vi "test - clear JKI String Queue Error.vi"(8 "error in (no error)":errorcluster, 11 "TestCase in":refnum<class "testcase-Basic-Function.lvclass">) -> (0 "error out":errorcluster, 3 "TestCase out":refnum<class "testcase-Basic-Function.lvclass">)   [LabVIEW 2017, in "testcase-Basic-Function.lvclass"]
uses:
  testcase-Basic-Function.lvclass
  161a5074-68cb-42ac-bbbd-290e101bf616.vi
  src/user.lib/_NEVSTOP/Communicable State Machine(CSM)/AdvanceAPI/CSM - Revert Arguments-Safe String.vi
  src/user.lib/_NEVSTOP/Communicable State Machine(CSM)/_Shared/Trim Single-line Text.vi
  src/user.lib/_NEVSTOP/Communicable State Machine(CSM)/AdvanceAPI/CSM - Make String Arguments Safe.vi
  src/user.lib/_NEVSTOP/Communicable State Machine(CSM)/AdvanceAPI/CSM - Break Down Multiple States String.vi
  src/user.lib/_NEVSTOP/Communicable State Machine(CSM)/AdvanceAPI/CSM - Compact Multiple States.vi
  src/user.lib/_NEVSTOP/Communicable State Machine(CSM)/AdvanceAPI/CSM - Keywords.vi
  <vilib>/addons/_JKI Toolkits/VI Tester/TestCase.llb/TestCase.lvclass
  src/user.lib/_NEVSTOP/Communicable State Machine(CSM)/Communicable State Machine.lvlib
  C:/Program Files (x86)/National Instruments/LabVIEW 2017/vi.lib/addons/_JKI Toolkits/VI Tester/TestCase.llb/TestCase.lvclass
panel:
  out "error in CSM":errorcluster
  in  "x":bool
  out "error for return":errorcluster
  out "State History":string
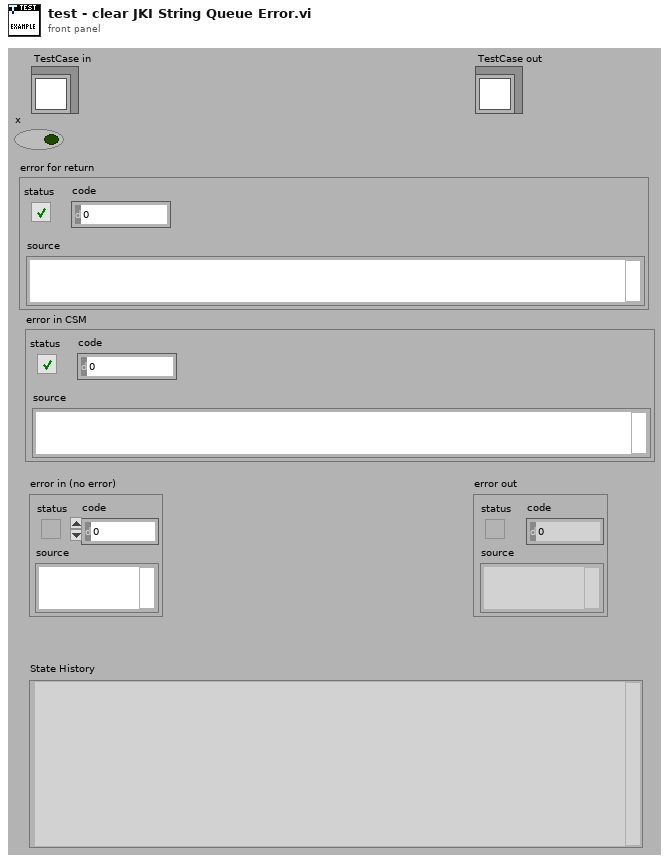
[diagram p1: front panel]
types:
  T1 = enum32{"Invalid", "Standard", "Closed", "Hidden", "Minimized", "Maximized"}
  T2 = enum32{"invalid app kind", "Development System", "Run Time System", "Student Edition", "Embedded LabVIEW", "Evaluation", "Custom"}
  T3 = typedef "Communicable State Machine.lvlib/_CSM_Response Source Message.ctl" = cluster{"‘State":string, "’Arguments":string, "’Error":errorcluster}
  T4 = cluster{"Current VI Reference":refnum<vi>, "Close Panel on Exit?":bool}
  T5 = cluster{"Core":cluster{"Current VI Reference":refnum<vi>, "Close Panel on Exit?":bool}, "Your Boolean data":bool, "Your string data":string}
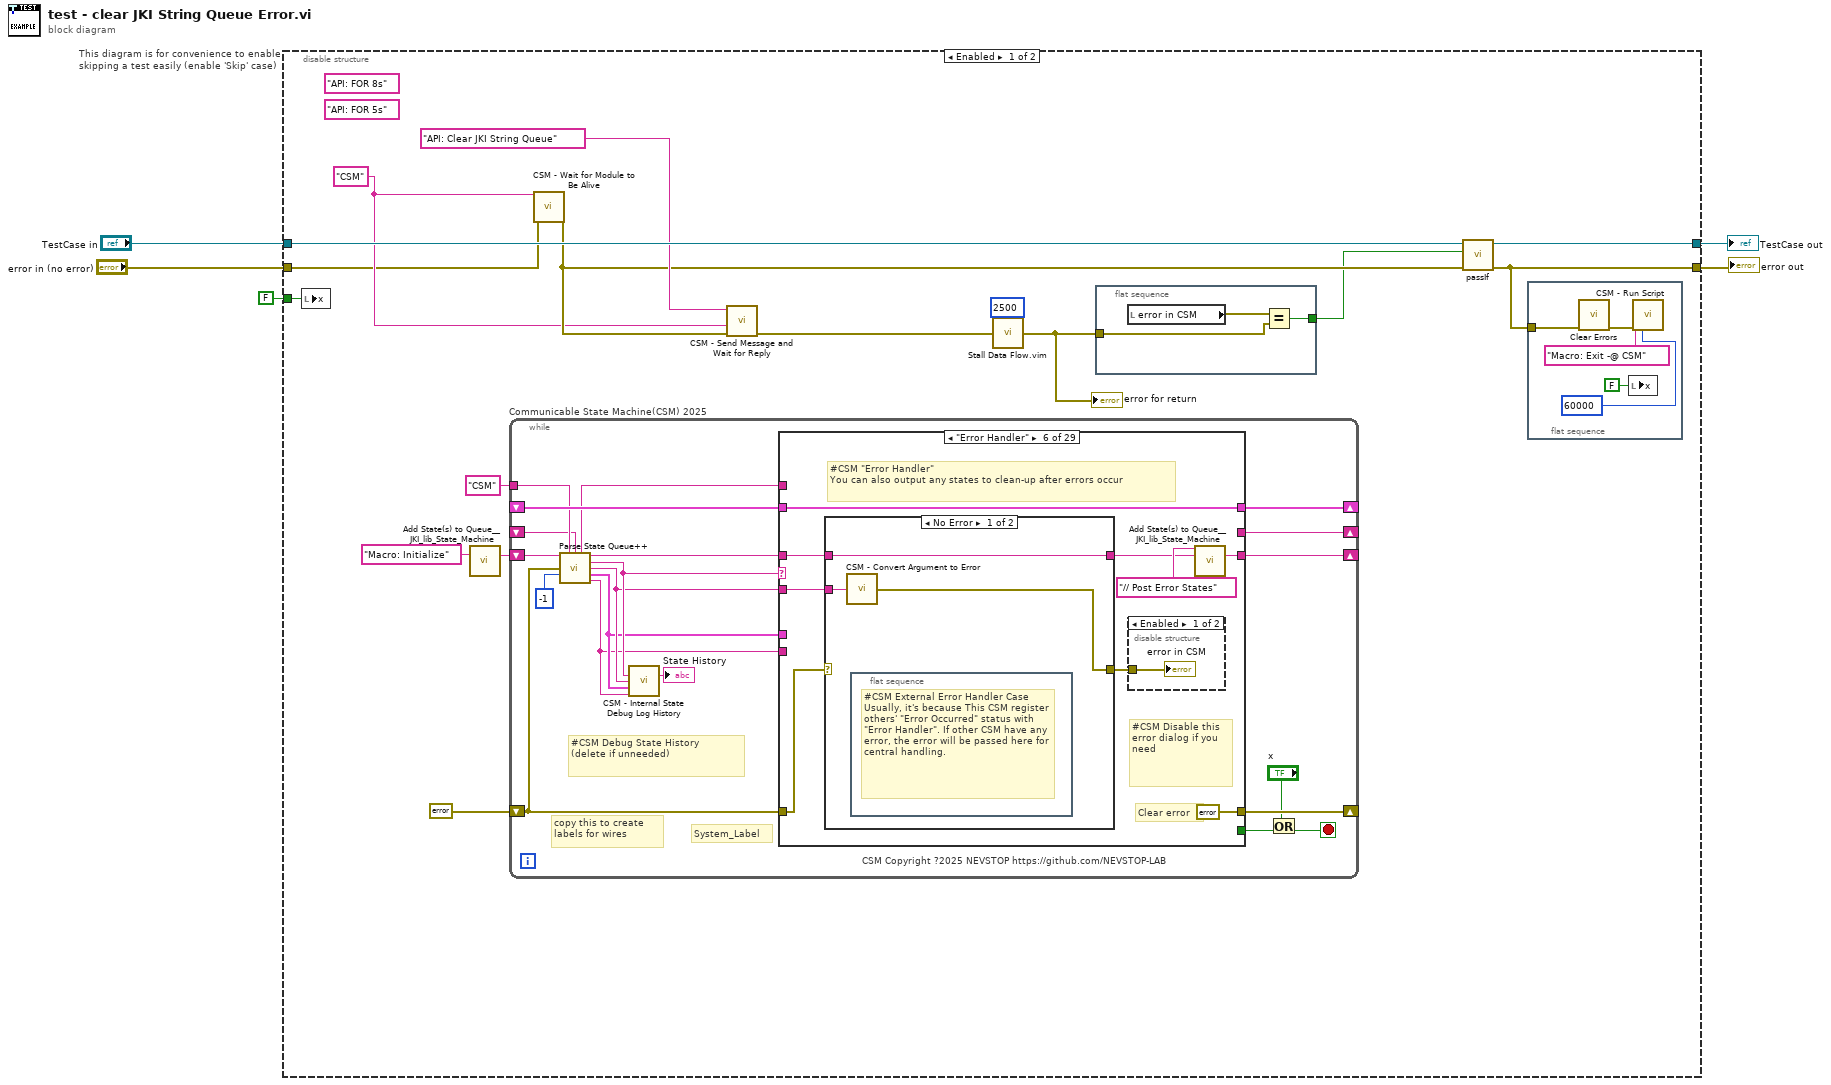
[diagram p0: block diagram]
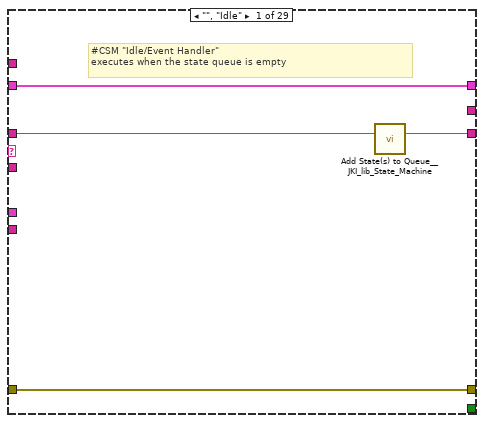
[diagram p2: hidden frame]
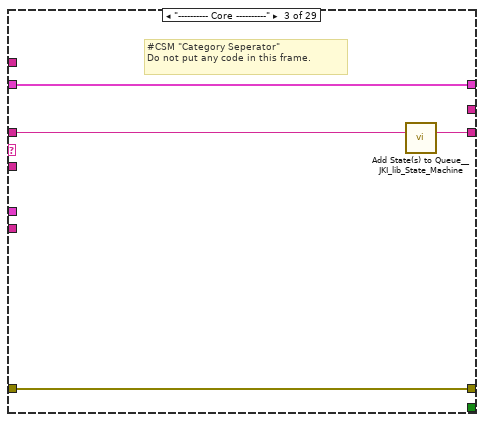
[diagram p4: hidden frame]
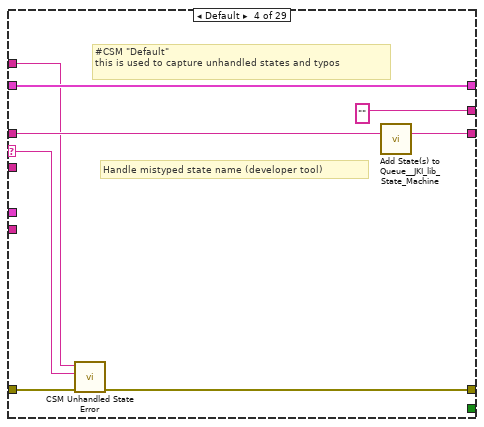
[diagram p5: hidden frame]
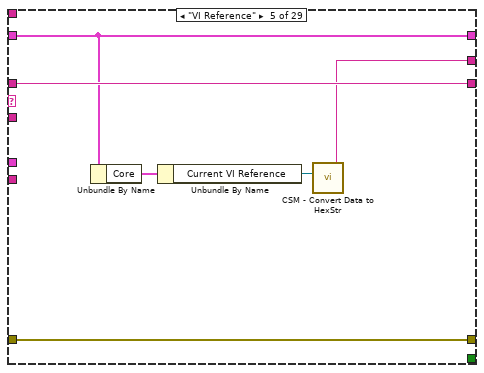
[diagram p6: hidden frame]
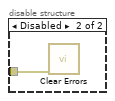
[diagram p7: hidden frame]
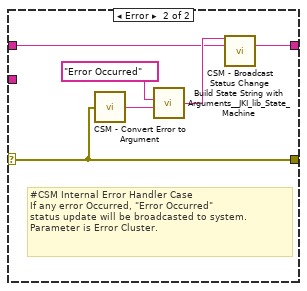
[diagram p8: hidden frame]
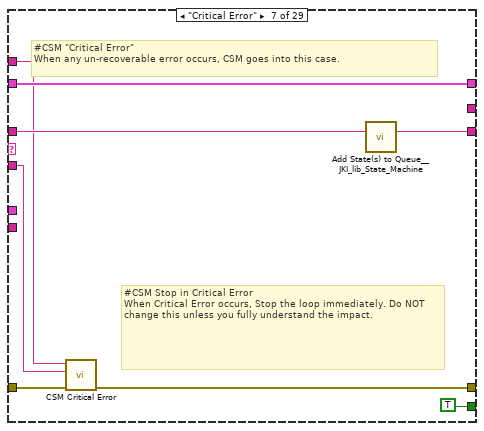
[diagram p9: hidden frame]
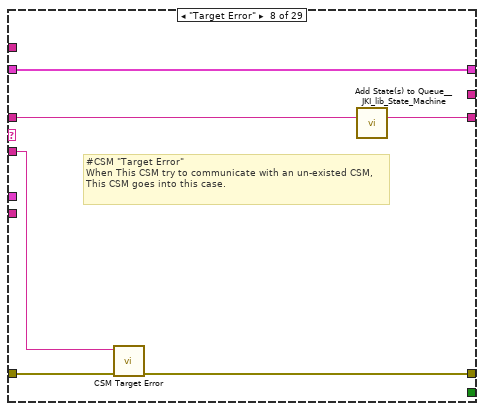
[diagram p10: hidden frame]
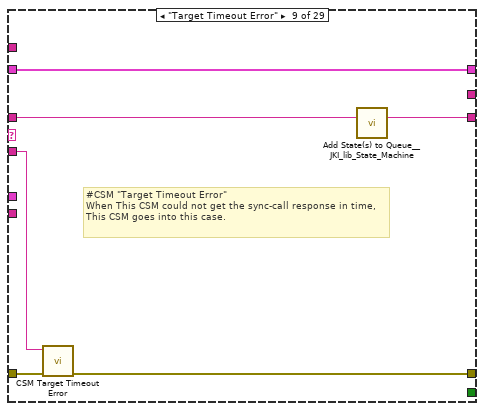
[diagram p11: hidden frame]
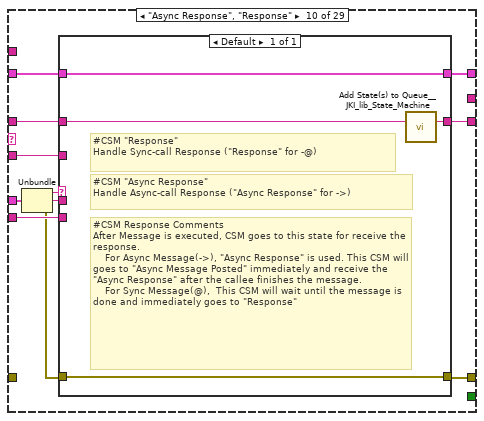
[diagram p12: hidden frame]
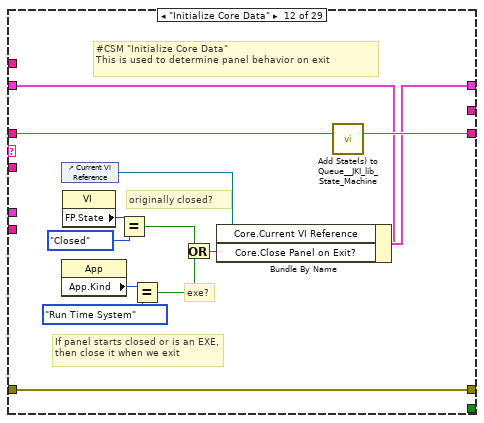
[diagram p14: hidden frame]
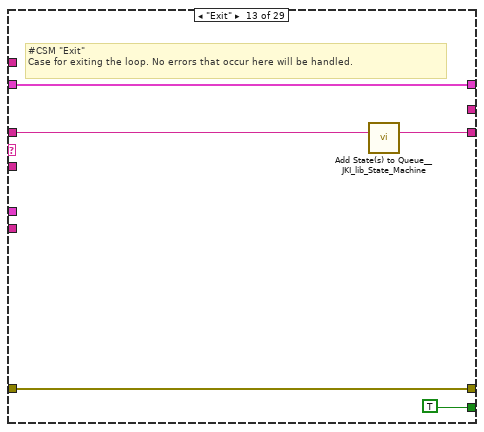
[diagram p15: hidden frame]
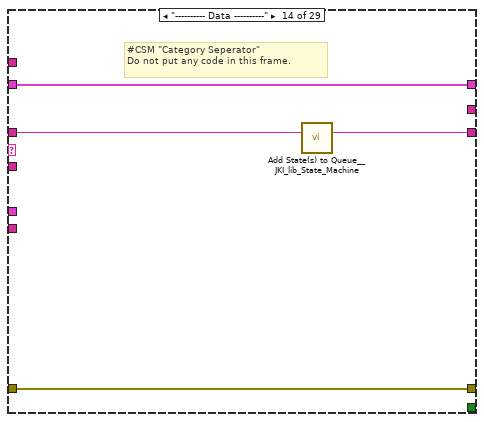
[diagram p16: hidden frame]
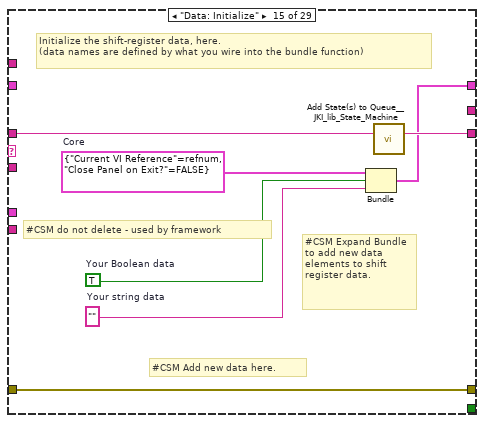
[diagram p17: hidden frame]
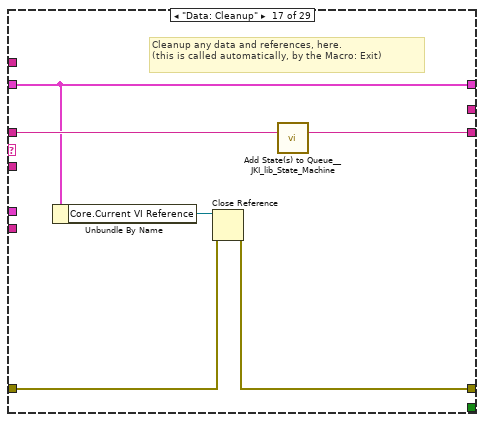
[diagram p19: hidden frame]
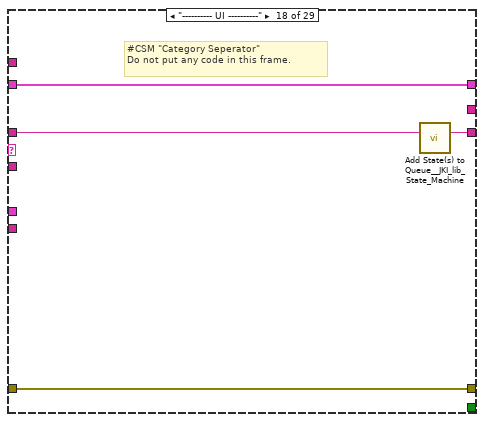
[diagram p20: hidden frame]
diagram:
  n1 = disable-structure "This diagram is for convenience to enable skipping a test easily (enable 'Skip' case)" shown="Enabled" {
    disable-tunnel: "TestCase in" -> [w15 w301]
    disable-tunnel: [w17 w299] -> w2
    disable-tunnel: [w16 w300] -> w4
    disable-tunnel: "error in (no error)" -> [w11 w298]
    disable-tunnel: FALSE ("x") -> [w8 _]
    frame Enabled {
      (unwired) "API: FOR 8s" ("State")
      (unwired) "API: FOR 5s" ("State")
      w12 = "CSM" ("Name (\"\" to Use UUID)")
      n2 = local write "x"(w8) -> ()
      n3 = call <vilib>:"Add State(s) to Queue__JKI_lib_State_Machine.vi"("State(s) in (\"\")"="Macro: Initialize" ("Init State(\"Macro: Initialize\")")) -> ("States Out"=w21:string)  [unwired: 14 in]
      n4 = while "Communicable State Machine(CSM) 2025" {
        shift-right: [w44] -> _
        shift-left: _ -> [w43]
        shift-right: [w47] -> _
        shift-left: errorcluster {"status"=FALSE, "code"=0, "source"=""} ("error out") -> [w42]
        shift-right: [w46] -> _
        shift-left: w21 -> [w48]
        tunnel: "CSM" ("Name (\"\" to Use UUID)") -> [w40]
        shift-right: [w41] -> _
        shift-left: _ -> [w34]
        stop <- w31 stop-if-true
        # "#CSM Debug State History\n(delete if unneeded)"
        # "copy this to create labels for wires"
        # "System_Label"
        # "CSM Copyright ?2025 NEVSTOP https://github.com/NEVSTOP-LAB"
        n5 = call "Parse State Queue++.vi"("State Queue"=w48, "Name (\"\" to Use UUID)"=w40, "Response Arguments"=w34, "Previous Error"=w42, "Dequeue (1 ms)"=-1 ("Timeout")) -> ("Name Used"=w35:string, "Remaining States"=w49:string, "Current State"=w39:string, "Arguments"=w38:string, "Additional Information"=w37:T3, "Source CSM"=w36:string)  [unwired: 5 in]
        n6 = call "CSM - Internal State Debug Log History.vi"("State"=w39, "Arguments (\"\")"=w38, ">> Response Source Message >>"=w37, "Source (\"\")"=w36) -> ("Debug Log"=→"State History":string)  [unwired: 11 in]
        n7 = case shown="\"Error Handler\"" w39 {
          selector: w39 -> [_ _ _ w63 _ _ _ _ _ _ _ _ _ _ _ _ _ _ _ _ _ _ _ _ _ _ _ _ _]
          tunnel: w49 -> [w50 w55 w60 w67 w73 w79 w100 w106 w112 w120 w131 w145 w150 w154 w161 w163 w170 w174 w178 w184 w199 w268 w273 w280 w282 _ w289 w293 w297]
          tunnel: w38 -> [_ _ _ _ _ w78 w96 w105 w110 w119 _ _ _ _ _ _ _ _ _ w179 w193 _ _ _ _ _ _ _ _]
          tunnel: w43 -> [w51 w54 w57 w65 w72 w82 w101 w107 w113 w122 w130 w138 w148 w151 _ w162 w165 w171 w176 w182 w195 w265 w270 w277 w281 w284 w286 w290 w294]
          tunnel: [w52 w56 w58 w61 w74 errorcluster {"status"=FALSE, "code"=0, "source"=""} ("error out") w97 w103 w109 w125 w132 w142 w147 w152 w158 w164 w166 w172 w175 w180 w196 w266 w271 w278 w283 w285 w287 w291 w295] -> w47
          tunnel: w42 -> [w52 w56 w58 w68 w74 w80 w102 w104 w111 _ w132 w142 w147 w152 w158 w164 w167 w172 w175 w181 w197 w266 w271 w278 w283 w285 w287 w291 w295]
          tunnel: [w53 w55 w59 w66 w73 w75 w99 w108 w114 w121 w131 w144 w149 w153 w160 w163 w169 w173 w177 w183 w198 w267 w272 w279 w282 _ w288 w292 w296] -> w46
          tunnel: [_ _ _ _ _ _ TRUE _ _ _ _ _ TRUE _ _ _ _ _ _ _ _ _ _ _ _ _ _ _ _] -> w45
          tunnel: [w51 w54 w57 w65 w72 w82 w101 w107 w113 w123 w130 w143 w148 w151 w159 w162 w165 w171 w176 w182 w195 w265 w270 w277 w281 w284 w286 w290 w294] -> w44
          tunnel: w36 -> [_ _ _ _ _ _ _ _ _ w117 _ _ _ _ _ _ _ _ _ _ _ _ _ _ _ _ _ _ _]
          tunnel: w37 -> [_ _ _ _ _ _ _ _ _ w124 _ _ _ _ _ _ _ _ _ _ _ _ _ _ _ _ _ _ _]
          tunnel: [_ _ _ "" w69 _ _ _ _ _ _ _ _ _ _ _ _ _ _ _ _ _ _ _ _ _ _ _ _] -> w41
          tunnel: w35 -> [_ _ _ w62 _ _ w95 _ _ _ _ _ _ _ _ _ _ _ _ _ _ _ _ _ _ _ _ _ _]
          frame "", "Idle" {
            # "#CSM \"Idle/Event Handler\"\nexecutes when the state queue is empty"
            n8 = call <vilib>:"Add State(s) to Queue__JKI_lib_State_Machine.vi"("State(s) in (\"\")"=w50) -> ("States Out"=w53:string)  [unwired: 14 in]
          }
          frame "CSM Documentation" {
            # "#CSM README FIRST\n\nCommunicable State Machine(CSM) is a LabVIEW application framework that builds upon JKI State Machine(JKISM). It follows the pattern of JKISM and extends the keywords to describe message communication between modules, including concepts such as Sync-Message, Async-Message, Subscription/Unsubscription of status - essential elements for creating reusable code modules. For more information, please visit the CSM wiki: https://nevstop-lab.github.io/CSM-Wiki/\n\nFor instructions on JKI State Machine, visit: http://jki.net/state-machine/\nFor information about CSM, visit: https://github.com/NEVSTOP-LAB"
            # "#CSM \"Documentation\"\nCase for holding CSM Documenation"
          }
          frame "---------- Core ----------" {
            # "#CSM \"Category Seperator\"\nDo not put any code in this frame."
            n9 = call <vilib>:"Add State(s) to Queue__JKI_lib_State_Machine.vi"("State(s) in (\"\")"=w60) -> ("States Out"=w59:string)  [unwired: 14 in]
          }
          frame Default {
            # "#CSM \"Default\"\nthis is used to capture unhandled states and typos"
            # "Handle mistyped state name (developer tool)"
            n10 = call "CSM Unhandled State Error.vi"("error in (no error)"=w68, "Undefined State"=w63, "CSM Name"=w62) -> ("error out"=w61:errorcluster)  [unwired: 8 in]
            n11 = call <vilib>:"Add State(s) to Queue__JKI_lib_State_Machine.vi"("State(s) in (\"\")"=w67) -> ("States Out"=w66:string)  [unwired: 14 in]
          }
          frame "VI Reference" {
            n12 = Unbundle By Name(w72) -> ("Core"=w71:T4)
            n13 = Unbundle By Name(w71) -> ("Current VI Reference"=w70:refnum<vi>)
            n14 = call "CSM - Convert Data to HexStr.vi"("Variant"=w70) -> ("HEX String (0-9,A-F)"=w69:string)  [unwired: 8 in]
          }
          frame "Error Handler" {
            # "#CSM Disable this error dialog if you need"
            # "#CSM \"Error Handler\"\nYou can also output any states to clean-up after errors occur"
            # "Clear error"
            n15 = case shown="No Error" w80 {
              selector: w80 -> [_ w89]
              tunnel: [w88 w91] -> w76
              tunnel: w79 -> [w88 w90]
              tunnel: w78 -> [w87 _]
              tunnel: [w86 w89] -> w81
              frame No Error {
                n16 = call "CSM - Convert Argument to Error.vi"("Argument"=w87) -> ("Error"=w86:errorcluster)  [unwired: 4 in]
                n17 = flat-sequence {
                  frame #0 {
                    # "#CSM External Error Handler Case\nUsually, it's because This CSM register others' \"Error Occurred\" status with \"Error Handler\". If other CSM have any error, the error will be passed here for central handling."
                  }
                }
              }
              frame Error {
                # "#CSM Internal Error Handler Case \nIf any error Occurred, \"Error Occurred\" \nstatus update will be broadcasted to system.\nParameter is Error Cluster."
                n18 = call "CSM - Convert Error to Argument.vi"("Error"=w89) -> ("Argument"=w93:string)  [unwired: 4 in]
                n19 = call <vilib>:"Build State String with Arguments__JKI_lib_State_Machine.vi"("Arguments (\"\")"=w93, "State"="Error Occurred" ("Status with Arguments")) -> ("State with Arguments"=w92:string)  [unwired: 4 in]
                n20 = call "CSM - Broadcast Status Change.vi"("Status With Arguments"=w92, "State Queue"=w90) -> ("Remaining States"=w91:string)  [unwired: 13 in]
              }
            }
            n21 = disable-structure shown="Enabled" {
              disable-tunnel: w81 -> [w84 w85]
              frame Enabled {
                "error in CSM" <- w84
              }
              frame Disabled {
                n22 = call <vilib>:"Clear Errors.vi"("error in (no error)"=w85) -> ()  [unwired: 5 in, 2 out]
              }
            }
            n23 = call <vilib>:"Add State(s) to Queue__JKI_lib_State_Machine.vi"("State(s) in Front (\"\")"="// Post Error States", "State(s) in (\"\")"=w76) -> ("States Out"=w75:string)  [unwired: 13 in]
          }
          frame "Critical Error" {
            # "#CSM Stop in Critical Error\nWhen Critical Error occurs, Stop the loop immediately. Do NOT change this unless you fully understand the impact."
            # "#CSM \"Critical Error\"\nWhen any un-recoverable error occurs, CSM goes into this case."
            n24 = call "CSM Critical Error.vi"("error in (no error)"=w102, "Arugments (As Reason)"=w96, "CSM Name"=w95) -> ("error out"=w97:errorcluster)  [unwired: 8 in]
            n25 = call <vilib>:"Add State(s) to Queue__JKI_lib_State_Machine.vi"("State(s) in (\"\")"=w100) -> ("States Out"=w99:string)  [unwired: 14 in]
          }
          frame "Target Error" {
            # "#CSM \"Target Error\"\nWhen This CSM try to communicate with an un-existed CSM, This CSM goes into this case."
            n26 = call "CSM Target Error.vi"("error in (no error)"=w104, "Arguments (As CSM Name)"=w105) -> ("error out"=w103:errorcluster)  [unwired: 9 in]
            n27 = call <vilib>:"Add State(s) to Queue__JKI_lib_State_Machine.vi"("State(s) in (\"\")"=w106) -> ("States Out"=w108:string)  [unwired: 14 in]
          }
          frame "Target Timeout Error" {
            # "#CSM \"Target Timeout Error\"\nWhen This CSM could not get the sync-call response in time, This CSM goes into this case."
            n28 = call "CSM Target Timeout Error.vi"("error in (no error)"=w111, "Arguments (As CSM Name)"=w110) -> ("error out"=w109:errorcluster)  [unwired: 9 in]
            n29 = call <vilib>:"Add State(s) to Queue__JKI_lib_State_Machine.vi"("State(s) in (\"\")"=w112) -> ("States Out"=w114:string)  [unwired: 14 in]
          }
          frame "Async Response", "Response" {
            n30 = Unbundle(w124) -> ("‘State"=w118:string, "’Arguments"=w116:string, "’Error"=w115:errorcluster)
            n31 = case shown="Default" w118 {
              tunnel: [w129] -> w125
              tunnel: w115 -> [w129]
              tunnel: [w128] -> w123
              tunnel: w122 -> [w128]
              tunnel: [w126] -> w121
              tunnel: w120 -> [w127]
              tunnel: w119 -> [_]
              tunnel: w117 -> [_]
              tunnel: w116 -> [_]
              frame Default {
                # "#CSM Response Comments\nAfter Message is executed, CSM goes to this state for receive the response.\n    For Async Message(->), \"Async Response\" is used. This CSM will goes to \"Async Message Posted\" immediately and receive the \"Async Response\" after the callee finishes the message.\n    For Sync Message(@),  This CSM will wait until the message is done and immediately goes to \"Response\""
                # "#CSM \"Async Response\"\nHandle Async-call Response (\"Async Response\" for ->)"
                # "#CSM \"Response\"\nHandle Sync-call Response (\"Response\" for -@)"
                n32 = call <vilib>:"Add State(s) to Queue__JKI_lib_State_Machine.vi"("State(s) in (\"\")"=w127) -> ("States Out"=w126:string)  [unwired: 14 in]
              }
            }
          }
          frame "Async Message Posted" {
            # "#CSM \"Async Message Posted\"\nAfter Async Message is posted (-> or ->| ), CSM goes to this state for post-action.\nYou can use Argument - State to tell which Async Message is called."
          }
          frame "Initialize Core Data" {
            # "#CSM \"Initialize Core Data\"\nThis is used to determine panel behavior on exit"
            # "originally closed?"
            # "exe?"
            # "If panel starts closed or is an EXE, then close it when we exit"
            n33 = control-ref of="Current VI Reference"() -> (w136:refnum<vi>)
            n34 = property class="App"() -> ("App.Kind"=w141:T2)  [unwired: 2 in, 2 out]
            n35 = property class="VI"() -> ("FP.State"=w135:T1)  [unwired: 2 in, 2 out]
            n36 = Equal?(x=w135, y=T1."Closed" ("Front Panel Window:State")) -> (x = y?=w133:bool)
            n37 = Equal?(x=w141, y=T2."Run Time System" ("Application:Kind")) -> (x = y?=w139:bool)
            n38 = Or(x=w133, y=w139) -> (x .or. y?=w137:bool)
            n39 = Bundle By Name(cluster=w138, "Core.Current VI Reference"=w136, "Core.Close Panel on Exit?"=w137) -> (w143:T5)
            n40 = call <vilib>:"Add State(s) to Queue__JKI_lib_State_Machine.vi"("State(s) in (\"\")"=w145) -> ("States Out"=w144:string)  [unwired: 14 in]
          }
          frame "Exit" {
            # "#CSM \"Exit\"\nCase for exiting the loop. No errors that occur here will be handled."
            n41 = call <vilib>:"Add State(s) to Queue__JKI_lib_State_Machine.vi"("State(s) in (\"\")"=w150) -> ("States Out"=w149:string)  [unwired: 14 in]
          }
          frame "---------- Data ----------" {
            # "#CSM \"Category Seperator\"\nDo not put any code in this frame."
            n42 = call <vilib>:"Add State(s) to Queue__JKI_lib_State_Machine.vi"("State(s) in (\"\")"=w154) -> ("States Out"=w153:string)  [unwired: 14 in]
          }
          frame "Data: Initialize" {
            w155 = T4 {"Current VI Reference"=refnum, "Close Panel on Exit?"=FALSE}  # Core
            w157 = TRUE  # Your Boolean data
            w156 = ""  # Your string data
            # "#CSM do not delete - used by framework"
            # "#CSM Expand Bundle to add new data elements to shift register data."
            # "#CSM Add new data here."
            # "Initialize the shift-register data, here.\n(data names are defined by what you wire into the bundle function)"
            n43 = Bundle("Core"=w155, "Your Boolean data"=w157, "Your string data"=w156) -> (w159:T5)  [unwired: 1 in]
            n44 = call <vilib>:"Add State(s) to Queue__JKI_lib_State_Machine.vi"("State(s) in (\"\")"=w161) -> ("States Out"=w160:string)  [unwired: 14 in]
          }
          frame "Data: Update Indicators" {
          }
          frame "Data: Cleanup" {
            # "Cleanup any data and references, here.\n(this is called automatically, by the Macro: Exit)"
            n45 = Unbundle By Name(w165) -> ("Core.Current VI Reference"=w168:refnum<vi>)
            n46 = Close Reference(reference=w168, error in (no error)=w167) -> (error out=w166:errorcluster)
            n47 = call <vilib>:"Add State(s) to Queue__JKI_lib_State_Machine.vi"("State(s) in (\"\")"=w170) -> ("States Out"=w169:string)  [unwired: 14 in]
          }
          frame "---------- UI ----------" {
            # "#CSM \"Category Seperator\"\nDo not put any code in this frame."
            n48 = call <vilib>:"Add State(s) to Queue__JKI_lib_State_Machine.vi"("State(s) in (\"\")"=w174) -> ("States Out"=w173:string)  [unwired: 14 in]
          }
          frame "UI: Initialize" {
            # "#CSM \"UI: Initialize\"\nInitialize the User Interface, here.\n(this is called automatically, by the Macro: Init)"
            n49 = call <vilib>:"Add State(s) to Queue__JKI_lib_State_Machine.vi"("State(s) in (\"\")"=w178) -> ("States Out"=w177:string)  [unwired: 14 in]
          }
          frame "UI: Cursor Set" {
            # "#CSM \"UI: Cursor Set\"\nSet and Unset Cursor Busy.\n(Usage: \"UI: Cursor Set >> Busy|Idle\")"
            # "Argument"
            n50 = disable-structure shown="TARGET_TYPE!=Windows" {
              disable-tunnel: w181 -> [w187 w192]
              disable-tunnel: [w186 w192] -> w180
              disable-tunnel: w179 -> [w185 _]
              frame condition #0 (active) {
                n51 = case shown="\"Idle\", Default" w185 {
                  tunnel: w187 -> [w189 w191]
                  tunnel: [w188 w190] -> w186
                  frame "Idle", Default {
                    n52 = call <vilib>:"Unset Busy.vi"("error in (no error)"=w189) -> ("error out"=w188:errorcluster)  [unwired: 10 in]
                  }
                  frame "Busy" {
                    n53 = call <vilib>:"Set Busy.vi"("error in (no error)"=w191) -> ("error out"=w190:errorcluster)  [unwired: 9 in, 1 out]
                  }
                }
              }
              frame condition #1 {
              }
            }
            n54 = call <vilib>:"Add State(s) to Queue__JKI_lib_State_Machine.vi"("State(s) in (\"\")"=w184) -> ("States Out"=w183:string)  [unwired: 14 in]
          }
          frame "UI: Front Panel State" {
            # "#CSM \"UI: Front Panel State\"\nSet Front Panel Open or Closed\n(Usage: \"UI: Front Panel State >> Open|Close\")"
            # "Argument"
            n55 = Unbundle By Name(w195) -> ("Core.Current VI Reference"=w194:refnum<vi>)
            n56 = call <vilib>:"Add State(s) to Queue__JKI_lib_State_Machine.vi"("State(s) in (\"\")"=w199) -> ("States Out"=w198:string)  [unwired: 14 in]
            n57 = case shown="\"Close\", \"Closed\"" w193 {
              tunnel: w197 -> [w205 w220 w231 w244 w257]
              tunnel: [w207 w221 w233 w246 w259] -> w196
              tunnel: w194 -> [w206 w218 w232 w245 w258]
              frame "Open", "Standard", Default {
                w200 = T1."Standard" ("State")
                n58 = property class="VI"(reference=w206, error in=w205) -> (reference out=w203:refnum<vi>, error out=w204:errorcluster, "FP.State"=w202:T1)
                n59 = Not Equal?(x=w202, y=w200) -> (x != y?=w201:bool)
                n60 = case shown="True" w201 {
                  tunnel: [w211 w213] -> w207
                  tunnel: w204 -> [w210 w213]
                  tunnel: w203 -> [w209 _]
                  tunnel: w200 -> [w208 _]
                  frame True {
                    n61 = invoke class="VI" method="FP.Open"(reference=w209, error in=w210, "Activate"=TRUE, "State"=w208) -> (error out=w211:errorcluster)  [unwired: 1 in, 4 out]
                  }
                  frame False {
                  }
                }
              }
              frame "Close", "Closed" {
                n62 = property class="VI"(reference=w218, error in=w220) -> (reference out=w217:refnum<vi>, error out=w219:errorcluster, "FP.State"=w215:T1)
                n63 = Not Equal?(x=w215, y=T1."Closed" ("Front Panel Window:State")) -> (x != y?=w214:bool)
                n64 = case shown="False" w214 {
                  tunnel: [w222 w225] -> w221
                  tunnel: w219 -> [w222 w224]
                  tunnel: w217 -> [_ w223]
                  frame False {
                  }
                  frame True {
                    n65 = invoke class="VI" method="FP.Close"(reference=w223, error in=w224) -> (error out=w225:errorcluster)  [unwired: 1 in, 2 out]
                  }
                }
              }
              frame "Hidden", "Hide" {
                w226 = T1."Hidden" ("State")
                n66 = property class="VI"(reference=w232, error in=w231) -> (reference out=w229:refnum<vi>, error out=w230:errorcluster, "FP.State"=w228:T1)
                n67 = Not Equal?(x=w228, y=w226) -> (x != y?=w227:bool)
                n68 = case shown="True" w227 {
                  tunnel: [w237 w238] -> w233
                  tunnel: w230 -> [w236 w238]
                  tunnel: w229 -> [w235 _]
                  tunnel: w226 -> [w234 _]
                  frame True {
                    n69 = invoke class="VI" method="FP.Open"(reference=w235, error in=w236, "State"=w234) -> (error out=w237:errorcluster)  [unwired: 2 in, 4 out]
                  }
                  frame False {
                  }
                }
              }
              frame "Minimize", "Minimized" {
                w239 = T1."Minimized" ("State")
                n70 = property class="VI"(reference=w245, error in=w244) -> (reference out=w242:refnum<vi>, error out=w243:errorcluster, "FP.State"=w241:T1)
                n71 = Not Equal?(x=w241, y=w239) -> (x != y?=w240:bool)
                n72 = case shown="True" w240 {
                  tunnel: [w250 w251] -> w246
                  tunnel: w243 -> [w249 w251]
                  tunnel: w242 -> [w248 _]
                  tunnel: w239 -> [w247 _]
                  frame True {
                    n73 = invoke class="VI" method="FP.Open"(reference=w248, error in=w249, "State"=w247) -> (error out=w250:errorcluster)  [unwired: 2 in, 4 out]
                  }
                  frame False {
                  }
                }
              }
              frame "Maximize", "Maximized" {
                w252 = T1."Maximized" ("State")
                n74 = property class="VI"(reference=w258, error in=w257) -> (reference out=w255:refnum<vi>, error out=w256:errorcluster, "FP.State"=w254:T1)
                n75 = Not Equal?(x=w254, y=w252) -> (x != y?=w253:bool)
                n76 = case shown="True" w253 {
                  tunnel: [w263 w264] -> w259
                  tunnel: w256 -> [w262 w264]
                  tunnel: w255 -> [w261 _]
                  tunnel: w252 -> [w260 _]
                  frame True {
                    n77 = invoke class="VI" method="FP.Open"(reference=w261, error in=w262, "State"=w260) -> (error out=w263:errorcluster)  [unwired: 2 in, 4 out]
                  }
                  frame False {
                  }
                }
              }
            }
          }
          frame "---------- Macro ----------" {
            # "#CSM \"Category Seperator\"\nDo not put any code in this frame."
            n78 = call <vilib>:"Add State(s) to Queue__JKI_lib_State_Machine.vi"("State(s) in (\"\")"=w268) -> ("States Out"=w267:string)  [unwired: 14 in]
          }
          frame "Macro: Initialize" {
            # "#CSM \"Macro: Initialize\"\nInitialization Macro (This is called once, when the VI starts)"
            n79 = call <vilib>:"Add State(s) to Queue__JKI_lib_State_Machine.vi"("State(s) in Front (\"\")"="Data: Initialize\nInitialize Core Data\nData: Update Indicators", "State(s) in (\"\")"=w273) -> ("States Out"=w272:string)  [unwired: 13 in]
          }
          frame "Macro: Exit" {
            # "#CSM \"Macro: Exit\"\nExit Macro (This is called once, when the VI exits)"
            n80 = call <vilib>:"Add State(s) to Queue__JKI_lib_State_Machine.vi"("State(s) in Front (\"\")"="//Exit Sub-Modules ", "State(s) at Back (\"\")"="Data: Cleanup\nExit") -> ("States Out"=w275:string)  [unwired: 13 in]
            n81 = call <vilib>:"Add State(s) to Queue__JKI_lib_State_Machine.vi"("State(s) in Front (\"\")"=w275, "State(s) in (\"\")"=w280) -> ("States Out"=w279:string)  [unwired: 13 in]
          }
          frame "---------- API ----------" {
            # "#CSM \"Category Seperator\"\nDo not put any code in this frame."
          }
          frame "API: Clear JKI String Queue" {
          }
          frame "---------- Action ----------" {
            # "#CSM \"Category Seperator\"\nDo not put any code in this frame."
            n82 = call <vilib>:"Add State(s) to Queue__JKI_lib_State_Machine.vi"("State(s) in (\"\")"=w289) -> ("States Out"=w288:string)  [unwired: 14 in]
          }
          frame "Action: action1" {
            # "#CSM \"Internal State\"\nThis category is used for holding internal states"
            n83 = call <vilib>:"Add State(s) to Queue__JKI_lib_State_Machine.vi"("State(s) in (\"\")"=w293) -> ("States Out"=w292:string)  [unwired: 14 in]
          }
          frame "Action: action2" {
            # "#CSM \"Internal State\"\nThis category is used for holding internal states"
            n84 = call <vilib>:"Add State(s) to Queue__JKI_lib_State_Machine.vi"("State(s) in (\"\")"=w297) -> ("States Out"=w296:string)  [unwired: 14 in]
          }
        }
        n85 = Or(x="x", y=w45) -> (x .or. y?=w31:bool)
      }
      n86 = call "CSM - Wait for Module to Be Alive.vi"("CSM Name"=w12, "error in (no error)"=w11) -> ("error out"=w13:errorcluster)  [unwired: 11 in, 2 out]
      n87 = call "CSM - Send Message and Wait for Reply.vi"("Error In (No Error)"=w13, "Target Module"=w12, "State"="API: Clear JKI String Queue") -> ("error out"=w10:errorcluster)  [unwired: 6 in, 2 out]
      n88 = call "Stall Data Flow.vim"("value in"=w10, "milliseconds to wait"=u32 2500) -> ("value out"=w7:errorcluster)  [unwired: 1 out]
      "error for return" <- w7
      n89 = flat-sequence {
        tunnel: [w24] -> w9
        tunnel: w7 -> [w23]
        frame #0 {
          n90 = local read "error in CSM"() -> (w22:errorcluster)
          n91 = Equal?(x=w22, y=w23) -> (x = y?=w24:bool)
        }
      }
      n92 = call-dynamic "passIf.vi"("error in (no error)"=w13, "pass"=w9, "TestCase in"=w15) -> ("error out"=w16:errorcluster, "TestCase out"=w17:refnum<class "testcase-Basic-Function.lvclass">)  [unwired: 7 in]
      n93 = flat-sequence {
        tunnel: w16 -> [w29]
        frame #0 {
          n94 = call <vilib>:"Clear Errors.vi"("error in (no error)"=w29) -> ("error out"=w28:errorcluster)  [unwired: 5 in, 1 out]
          n95 = local write "x"(FALSE ("x")) -> ()
          n96 = call "CSM - Run Script.vi"("CSM Scripts"="Macro: Exit -@ CSM", "error in (no error)"=w28, "Response Timeout (-2 Using Global Settings)"=60000) -> ()  [unwired: 10 in, 3 out]
        }
      }
    }
    frame Disabled {
      # "skip test result while test is under development"
      n97 = call <vilib>:"skip.vi"("error in (no error)"=w298, "TestCase in"=w301) -> ("error out"=w300:errorcluster, "TestCase out"=w299:refnum<class "testcase-Basic-Function.lvclass">)  [unwired: 8 in]
    }
  }
  "error out" <- w4
  "TestCase out" <- w2
